vi "Read Image Header (SubVI).vi"(11 "File REF In":refnum<file>) -> (0 "Image Header":T1={"Image ID Code"=[175, 33, 9, 248], "Image Header Size"=1024, "Depth"=8, "N Channels"=1, "Num of Image Blocks"=69}, 3 "File REF Out":refnum<file>)   [LabVIEW 2015]
uses:
  Controls/Image Header.ctl
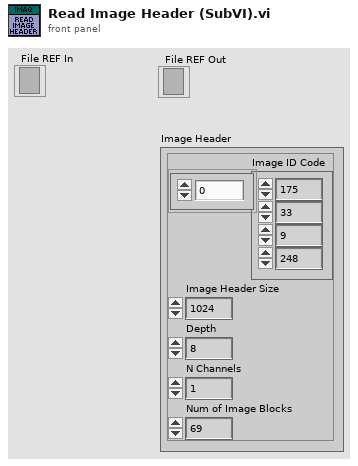
[diagram p1: front panel]
types:
  T1 = typedef "Image Header.ctl" = cluster{"Image ID Code":u8[], "Image Header Size":i32, "Depth":i32, "N Channels":i32, "Num of Image Blocks":i32}
  T2 = enum16{"big-endian, network order", "native, host order", "little-endian"}
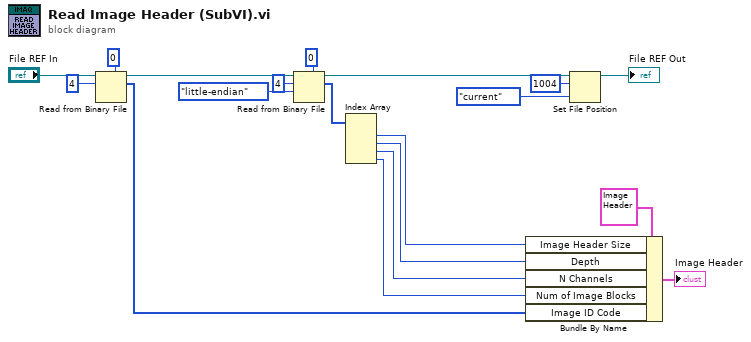
[diagram p0: block diagram]
diagram:
  n1 = Read from Binary File(5:u8 0, 10:4 ("count (1)"), 11:"File REF In") -> (2:w2:u8[], 3:w13:refnum<file>)  [unwired: 3 in, 2 out]
  n2 = Read from Binary File(5:0, 9:T2."little-endian" ("byte order (0:big-endian, network order)"), 10:4 ("count (1)"), 11:w13) -> (2:w14:i32[], 3:w18:refnum<file>)  [unwired: 2 in, 2 out]
  n3 = Index Array(array=w14) -> (element #1=w6:i32, element #2=w5:i32, element #3=w4:i32, element #4=w3:i32)  [unwired: 4 in]
  n4 = Bundle By Name(cluster=T1 {"Image ID Code"=[175, 33, 9, 248], "Image Header Size"=1024, "Depth"=8, "N Channels"=1, "Num of Image Blocks"=69}, "Image Header Size"=w6, "Depth"=w5, "N Channels"=w4, "Num of Image Blocks"=w3, "Image ID Code"=w2) -> (→"Image Header":T1)
  n5 = Set File Position(offset (in bytes) (0)=i64 1004, refnum=w18, from (0:start)=enum16{"start", "end", "current"}."current") -> (refnum out=→"File REF Out":refnum<file>)  [unwired: 1 in, 1 out]
